vi "Msg EnQ.vi"(9 "Priority?":bool, 10 "Msg":refnum<class "Msg.lvclass">, 11 "Msg Q in":refnum<class "Msg Q.lvclass">) -> (0 "error out":errorcluster)   [LabVIEW 2021, in "LVCAM.lvlib" / "Msg Q.lvclass"]
uses:
  Msg Q.lvclass
  Msg/Msg.lvclass
  Msg Q.lvclass/Msg Q.ctl
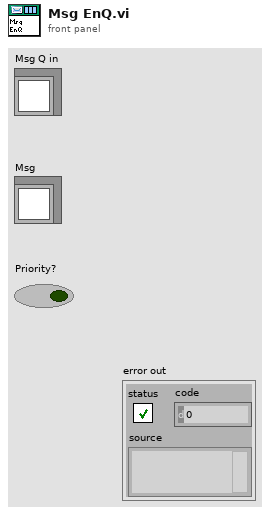
[diagram p1: front panel]
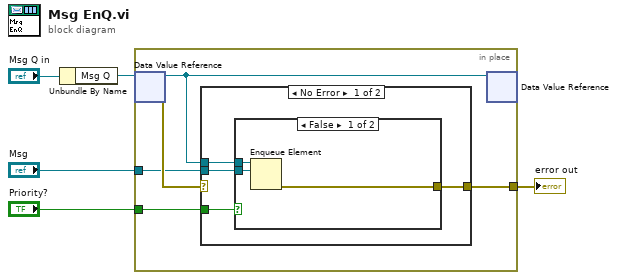
[diagram p0: block diagram]
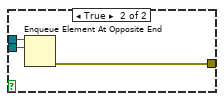
[diagram p2: hidden frame]
diagram:
  n1 = Unbundle By Name("Msg Q in") -> ("Msg Q"=w2:refnum<data-value>)
  n2 = in-place {
    in-place-border: [w9] -> w4
    in-place-border: "Msg" -> [w8]
    in-place-border: "Priority?" -> [w6]
    n3 = in-place-dvr #1(w2) -> (w7:refnum<queue>, w10:errorcluster)
    n4 = case shown="No Error" w10 {
      selector: w10 -> [_ w21]
      tunnel: [w14 w21] -> w9
      tunnel: w8 -> [w12 _]
      tunnel: w7 -> [w13 _]
      tunnel: w6 -> [w11 _]
      frame No Error {
        n5 = case shown="False" w11 {
          tunnel: [w17 w18] -> w14
          tunnel: w13 -> [w16 w20]
          tunnel: w12 -> [w15 w19]
          frame False {
            n6 = Enqueue Element(queue=w16, element=w15) -> (error out=w17:errorcluster)  [unwired: 2 in, 2 out]
          }
          frame True {
            n7 = Enqueue Element At Opposite End(queue=w20, element=w19) -> (error out=w18:errorcluster)  [unwired: 2 in, 2 out]
          }
        }
      }
      frame Error {
      }
    }
    n8 = in-place-dvr #1(w7) -> ()  [unwired: 2 out]
  }
  "error out" <- w4
